vi "Reference Object.vi"() -> ()   [LabVIEW 2023]
doc: "This example demonstrates Reference Class, a class that stores its data by reference. The data of Reference Class is an instance of Simple Class, a class that stores its data by value. Refer to the LabVIEW Help for more information about LabVIEW object-oriented programming."
uses:
  ReferenceClass/Reference Class.lvclass
  SimpleClass/Simple Class.lvclass
panel:
  out "on-off out":bool
  in  "on-off":bool=TRUE
  out "name out":string
  in  "name":string="test"
  # "Overview: Demonstrates a class that stores its data by reference rather than by value.\nInstructions:\nOpen the block diagram and refer to the comments there."
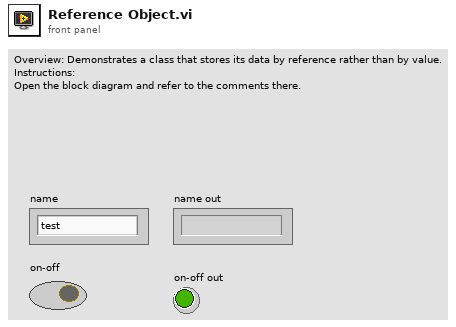
[diagram p1: front panel]
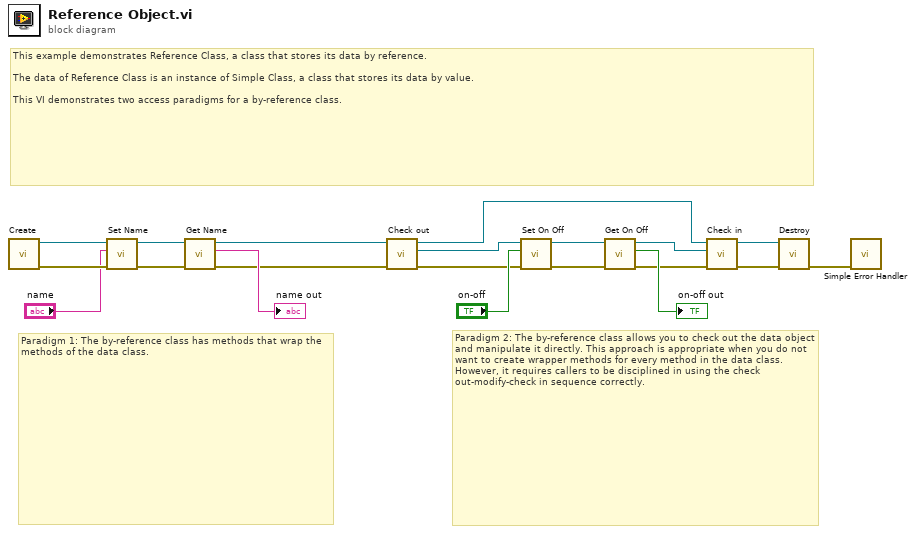
[diagram p0: block diagram]
diagram:
  # "This example demonstrates Reference Class, a class that stores its data by reference.\n\nThe data of Reference Class is an instance of Simple Class, a class that stores its data by value.\n\nThis VI demonstrates two access paradigms for a by-reference class."
  # "Paradigm 2: The by-reference class allows you to check out the data object and manipulate it directly. This approach is appropriate when you do not want to create wrapper methods for every method in the data class. However, it requires callers to be disciplined in using the check out-modify-check in sequence correctly."
  # "Paradigm 1: The by-reference class has methods that wrap the methods of the data class."
  n1 = call "Create.vi"() -> ("error out"=w20:errorcluster, "reference Class out"=w19:refnum<class "Reference Class.lvclass">)  [unwired: 10 in]
  n2 = call "Set Name.vi"("error in (no error)"=w20, "name"="name", "reference Class in"=w19) -> ("error out"=w15:errorcluster, "reference Class out"=w16:refnum<class "Reference Class.lvclass">)  [unwired: 7 in]
  n3 = call "Get Name.vi"("error in (no error)"=w15, "reference Class in"=w16) -> ("error out"=w9:errorcluster, "name"=→"name out":string, "reference Class out"=w10:refnum<class "Reference Class.lvclass">)  [unwired: 7 in]
  n4 = call "Check out.vi"("error in (no error)"=w9, "reference Class in"=w10) -> ("error out"=w7:errorcluster, "data"=w8:refnum<class "Simple Class.lvclass">, "reference Class out"=w6:refnum<class "Reference Class.lvclass">)  [unwired: 7 in]
  n5 = call "Set On Off.vi"("error in (no error)"=w7, "on-off"="on-off", "simple Class in"=w8) -> ("error out"=w12:errorcluster, "simple Class out"=w14:refnum<class "Simple Class.lvclass">)  [unwired: 7 in]
  n6 = call "Get On Off.vi"("error in (no error)"=w12, "simple Class in"=w14) -> ("error out"=w4:errorcluster, "on-off"=→"on-off out":bool, "simple Class out"=w5:refnum<class "Simple Class.lvclass">)  [unwired: 7 in]
  n7 = call "Check in.vi"("error in (no error)"=w4, "data"=w5, "reference Class in"=w6) -> ("error out"=w3:errorcluster, "reference Class out"=w2:refnum<class "Reference Class.lvclass">)  [unwired: 7 in]
  n8 = call "Destroy.vi"("error in (no error)"=w3, "reference Class in"=w2) -> ("error out"=w1:errorcluster)  [unwired: 8 in, 1 out]
  n9 = call <vilib>:"Simple Error Handler.vi"("error in (no error)"=w1) -> ()  [unwired: 4 in, 5 out]
